vi "sample_main_2.vi"() -> ()   [LabVIEW 2020]
panel:
  out "object":refnum<class>
  out "error out":errorcluster
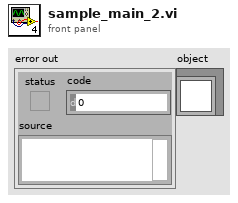
[diagram p1: front panel]
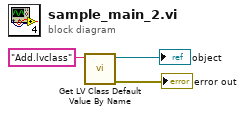
[diagram p0: block diagram]
diagram:
  n1 = call <vilib>:"Get LV Class Default Value By Name.vi"("class name"="Add.lvclass") -> ("error out"=→"error out":errorcluster, "object"=→"object":refnum<class>)  [unwired: 9 in]
